vi "SCC Close SCC Project.vi"(8 "error in (no error)":errorcluster, 11 "source control reference in":T1) -> (0 "error out":errorcluster, 2 "status message":string)   [LabVIEW 2017, in "NI_SCC.lvlib"]
doc: "Closes an existing source control reference."
uses:
  <vilib>/SourceControl/sccapi/NI_SCC.lvlib
  <vilib>/SourceControl/sccapi/SCCAPI Refnum.ctl
  <vilib>/SourceControl/sccapi/SCCAPI SCC Operations.ctl
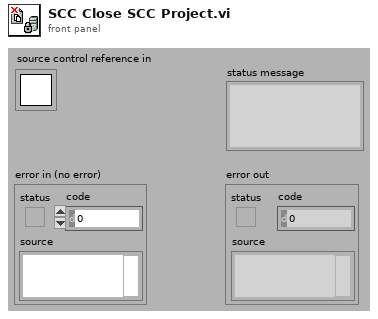
[diagram p1: front panel]
types:
  T1 = typedef "NI_SCC.lvlib/SCCAPI Refnum.ctl" = refnum<k1>
  T2 = typedef "NI_SCC.lvlib/SCCAPI SCC Operations.ctl" = enum16{"Add", "Check In", "Check Out", "Close Project", "Compare Files", "Compare VIs", "Configure Project", "File History", "File Properties", "File Status", "Find All Providers", "Get Advanced Command Options", "Get File Copy", "Get Latest Version", "Get Project Name", "Get StaticVI Path", "Initialize", "Not A Source Control Reference", "Open Project", "Provider Supports Functionality", "Remove", "Run Provider", "Undo Check Out", "Uninitialize", "Is File In Local Path"}
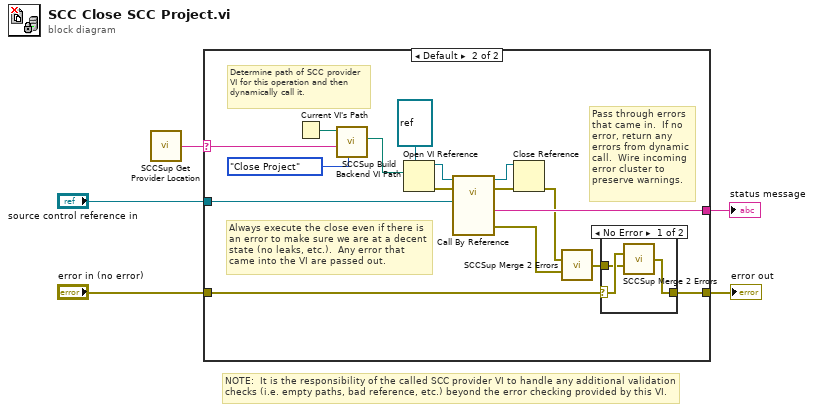
[diagram p0: block diagram]
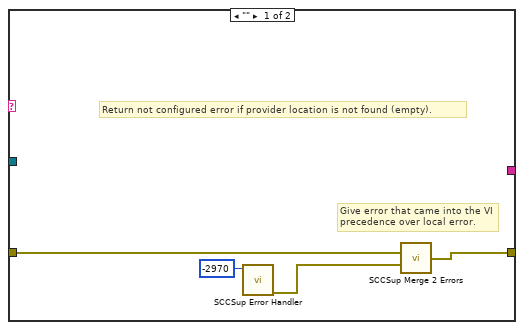
[diagram p2: hidden frame]
diagram:
  # "NOTE:  It is the responsibility of the called SCC provider VI to handle any additional validation checks (i.e. empty paths, bad reference, etc.) beyond the error checking provided by this VI."
  n1 = call <vilib>:"SCCSup Get Provider Location.vi"() -> ("provider location"=w1:string)  [unwired: 6 in]
  n2 = case shown="Default" w1 {
    selector: w1 -> [_ w13]
    tunnel: [w6 w17] -> w5
    tunnel: "source control reference in" -> [_ w25]
    tunnel: [_ w24] -> w4
    tunnel: "error in (no error)" -> [w8 w18]
    frame "" {
      # "Give error that came into the VI precedence over local error."
      # "Return not configured error if provider location is not found (empty)."
      n3 = call <vilib>:"SCCSup Error Handler.vi"("scc error code"=-2970 ("code")) -> ("error out"=w7:errorcluster)  [unwired: 10 in]
      n4 = call <vilib>:"SCCSup Merge 2 Errors.vi"("Error IO 1"=w8, "Error IO 2"=w7) -> ("Error IO out"=w6:errorcluster)  [unwired: 13 in]
    }
    frame Default {
      # "Pass through errors that came in.  If no error, return any errors from dynamic call.  Wire incoming error cluster to preserve warnings."
      # "Always execute the close even if there is an error to make sure we are at a decent state (no leaks, etc.).  Any error that came into the VI are passed out."
      # "Determine path of SCC provider VI for this operation and then dynamically call it."
      n5 = Current VI's Path() -> (path=w16:path)
      n6 = call <vilib>:"SCCSup Build Backend VI Path.vi"("scc operation"=SCCAPI_SCC_Operations."Close Project", "provider location"=w13, "caller path"=w16) -> ("scc backend VI path"=w15:path)  [unwired: 8 in]
      n7 = Open VI Reference(type specifier VI Refnum (for type only)=refnum<vi> refnum, vi path=w15) -> (vi reference=w22:refnum<vi>, error out=w21:errorcluster)  [unwired: 4 in]
      n8 = call-by-ref "?"(reference=w22, error in=w21, "source control reference in"=w25) -> (reference out=w20:refnum<vi>, error out=w19:errorcluster, 0:"error out"=w11:errorcluster, "status message"=w24:string)  [unwired: 9 in]
      n9 = Close Reference(reference=w20, error in (no error)=w19) -> (error out=w12:errorcluster)
      n10 = call <vilib>:"SCCSup Merge 2 Errors.vi"("Error IO 1"=w12, "Error IO 2"=w11) -> ("Error IO out"=w10:errorcluster)  [unwired: 13 in]
      n11 = case shown="No Error" w18 {
        selector: w18 -> [w27 w29]
        tunnel: [w28 w29] -> w17
        tunnel: w10 -> [w26 _]
        frame No Error {
          n12 = call <vilib>:"SCCSup Merge 2 Errors.vi"("Error IO 1"=w27, "Error IO 2"=w26) -> ("Error IO out"=w28:errorcluster)  [unwired: 13 in]
        }
        frame Error {
        }
      }
    }
  }
  "error out" <- w5
  "status message" <- w4
